vi "TrigGenEdgewave.vi"(8 "pt#":i32=40) -> (0 "Digital Waveform Graph":digitalwaveform(graph)={"t0"=timestamp(0 s since 1904-01-01), "dt"=0.025, "Y"={"transitions"=[], "data"=array5342x4[21368 elements]}}, 3 "delays":u32[](array[numeric])=[10, 197608, 262154, 0, 1, 1, 40, 1, 1, 278, 4000, 0, 0, 0, 0, 0, 0, 0, 0, 0, 0, 0, 0, 0, 0, 0, 0, 0, 0, 0, 0, 0, 0, 0, 0, 0, 0, 0, 0, 0])   [LabVIEW 2017]
uses:
  <vilib>/Waveform/DWDTOps.llb/DWDT Boolean Array to Digital.vi
panel:
  in  "pd delay":i16
  # "Show the timing diagram of laser or daq within one laser cycle"
  # "ignore the X time here, It is not right. find the right time in FPGA code\nOnly for you to see the timing"
  # "Note: 197608=3*2^16+1000"
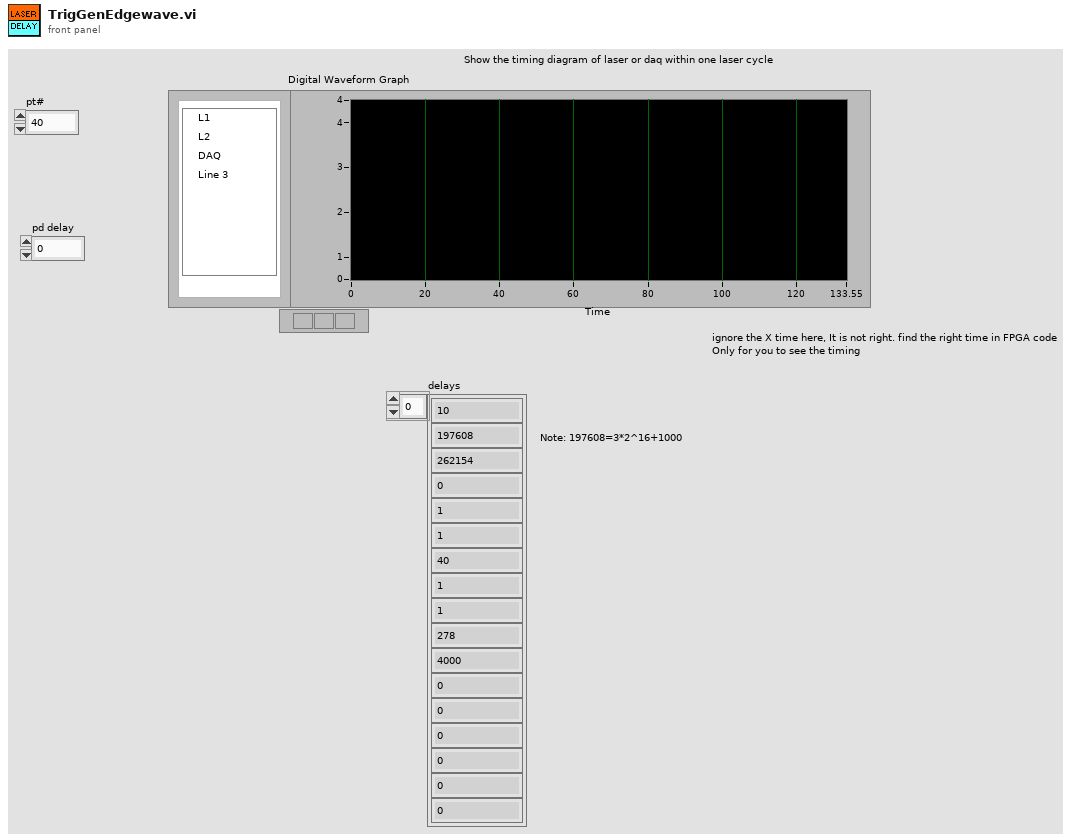
[diagram p1: front panel]
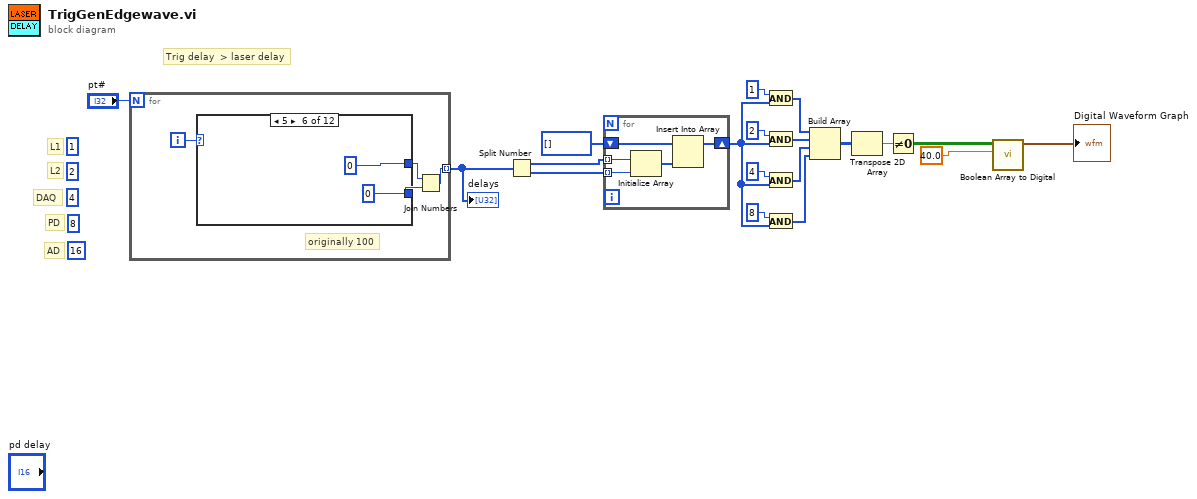
[diagram p0: block diagram]
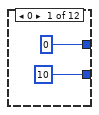
[diagram p2: hidden frame]
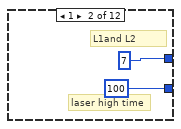
[diagram p3: hidden frame]
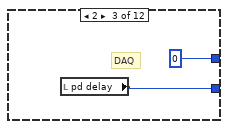
[diagram p4: hidden frame]
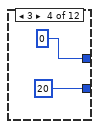
[diagram p5: hidden frame]
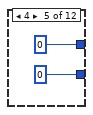
[diagram p6: hidden frame]
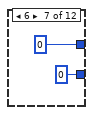
[diagram p7: hidden frame]
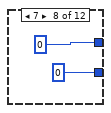
[diagram p8: hidden frame]
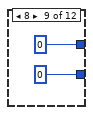
[diagram p9: hidden frame]
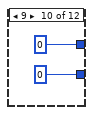
[diagram p10: hidden frame]
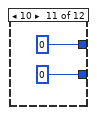
[diagram p11: hidden frame]
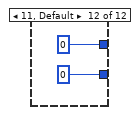
[diagram p12: hidden frame]
diagram:
  (unwired) u16 16
  (unwired) u16 8
  (unwired) u16 4
  (unwired) u16 2
  (unwired) u16 1
  # "Trig delay  > laser delay"
  # "AD"
  # "PD"
  # "DAQ"
  # "L2"
  # "L1"
  n1 = for {
    N: "pt#" -> [_]
    tunnel: [w22] -> w8 mode=indexing
    i -> [w23]
    # "originally 100"
    n2 = case shown="5" w23 {
      tunnel: [u16 0 ("element") u16 7 u16 0 u16 0 u16 0 ("pddelay") u16 0 u16 0 u16 0 u16 0 u16 0 ("pddelay") u16 0 ("pddelay") u16 0 ("pddelay")] -> w21
      tunnel: [u16 10 ("pddelay") u16 100 w28 u16 20 ("pddelay") u16 0 ("pddelay") u16 0 ("pddelay") u16 0 ("pddelay") u16 0 ("pddelay") u16 0 ("pddelay") u16 0 ("pddelay") u16 0 ("pddelay") u16 0 ("pddelay")] -> w20
      frame 0 {
      }
      frame 1 {
        # "laser high time"
        # "L1and L2"
      }
      frame 2 {
        # "DAQ"
        n3 = local read "pd delay"() -> (w28:i16)
      }
      frame 3 {
      }
      frame 4 {
      }
      frame 5 {
      }
      frame 6 {
      }
      frame 7 {
      }
      frame 8 {
      }
      frame 9 {
      }
      frame 10 {
      }
      frame 11, Default {
      }
    }
    n4 = Join Numbers(hi=w21, lo=w20) -> ((hi.lo)=w22:u32)
  }
  "delays" <- w8
  n5 = Split Number(x=w8) -> (hi(x)=w7:u16[], lo(x)=w6:u16[])
  n6 = for {
    tunnel: w6 -> [w52] mode=indexing
    tunnel: w7 -> [w51] mode=indexing
    shift-right: [w50] -> w2
    shift-left: u16[] [] -> [w49]
    n7 = Initialize Array(w51, w52) -> (w48:u16[])
    n8 = Insert Into Array(array=w49, new element=w48) -> (w50:u16[])  [unwired: 1 in]
  }
  n9 = And(x=u16 1, y=w2) -> (x .and. y?=w16:u16[])
  n10 = And(x=u16 2, y=w2) -> (x .and. y?=w15:u16[])
  n11 = And(x=u16 4, y=w2) -> (x .and. y?=w14:u16[])
  n12 = And(x=u16 8, y=w2) -> (x .and. y?=w1:u16[])
  n13 = Build Array(w16, w15, w14, w1) -> (w10:u16[][])
  n14 = Transpose 2D Array(2D array=w10) -> (transposed array=w9:u16[][])
  n15 = Not Equal To 0?(x=w9) -> (x != 0?=w13:bool[][])
  n16 = call-poly <vilib>:"Boolean Array to Digital.vi"("sample rate"=40.0, "boolean array"=w13) -> ("digital waveform"=→"Digital Waveform Graph":digitalwaveform)  [unwired: 8 in, 1 out]
